vi "Fpga.vi"() -> ()   [LabVIEW 2015]
uses:
  <vilib>/rvi/Emulation/niFpgaGetClockAttributes.vi
  <vilib>/rvi/Emulation/niFpgaSctlEmulationGetInTimedLoop.vi
  <vilib>/rvi/Emulation/niFpgaEmulationReportErrorSimple.vi
  <vilib>/rvi/eio/common/nirviEmuTemplateMethod_errors.vi
  <vilib>/rvi/Emulation/niFpgaCriticalErrorInLSC.vi
  <vilib>/rvi/interface/RandomDataEmulation/niFpgaRandomDataHandleErrors.vi
  <vilib>/eio/EIONode/EIONode.xnode
  <vilib>/rvi/DataTransferAndStorage/Container/XNode/niFpgaContainer.xnode
  <vilib>/rvi/interface/RandomDataEmulation/nirviRandomDataFpgaReadWriteTemplate.vi
panel:
  out "Timed Out?":bool
  out "Boolean 2":bool
  out "Mod3/AI0 2":fxp<+/-,16,5>
  in  "Mod4/AO0 2":i16
  out "x-y":u32
  out "Mod2/DIO6":bool
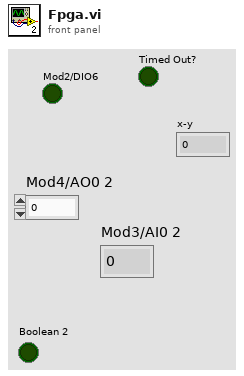
[diagram p1: front panel]
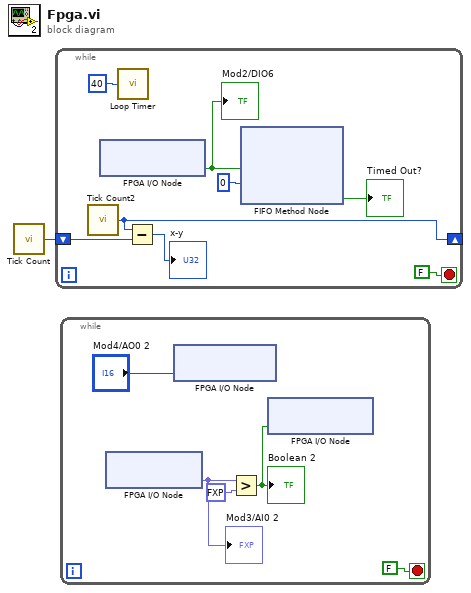
[diagram p0: block diagram]
diagram:
  n1 = call "Tick Count"() -> ("Tick Count(Ticks)"=w1:u32)
  n2 = while {
    shift-right: [w8] -> _
    shift-left: w1 -> [w7]
    stop <- FALSE stop-if-true
    n3 = call "Tick Count2"() -> ("Tick Count(Ticks)"=w8:u32)
    n4 = xnode "FPGA I/O Node"() -> ("Mod2/DIO6"=w5:bool)  [unwired: 1 in, 1 out]
    "Mod2/DIO6" <- w5
    n5 = call "Loop Timer"("Count(Ticks)"=u32 40) -> ()  [unwired: 1 out]
    n6 = Subtract(x=w8, y=w7) -> (x-y=→"x-y":u32)
    n7 = xnode ("FIFO Method Node")("Element"=w5, "Timeout"=0) -> ("Timed Out?"=→"Timed Out?":bool)  [unwired: 1 in, 1 out]
  }
  n8 = while {
    stop <- FALSE stop-if-true
    n9 = xnode "FPGA I/O Node"() -> ("Mod3/AI0"=w12:fxp<+/-,16,5>)  [unwired: 1 in, 1 out]
    "Mod3/AI0 2" <- w12
    n10 = xnode "FPGA I/O Node"("Mod4/AO0"="Mod4/AO0 2") -> ()  [unwired: 1 in, 1 out]
    n11 = Greater?(x=w12, y=fxp<+/-,16,5> 2.0) -> (0:w14:bool)
    "Boolean 2" <- w14
    n12 = xnode "FPGA I/O Node"("Mod2/DIO0"=w14) -> ()  [unwired: 1 in, 1 out]
  }
